vi "readFromXML.vi"(8 "error in (no error)":errorcluster, 10 "XML in":string, 11 "Ephemeris in":refnum<class "Ephemeris.lvclass">) -> (0 "error out":errorcluster, 3 "Ephemeris out":refnum<class "Ephemeris.lvclass">)   [LabVIEW 2022 SP3, in "TCSDataDefinitions.lvlib" / "TCSCommand.lvlib" / "TargetConfiguration.lvlib" / "Target.lvlib" / "Ephemeris.lvclass"]
uses:
  Ephemeris.lvclass
  Ephemeris.lvclass/Ephemeris.ctl
  Target/Target.lvclass
  <userlib>/Common/XML/XMLParser/XMLParser.lvclass
panel:
  out "file":string
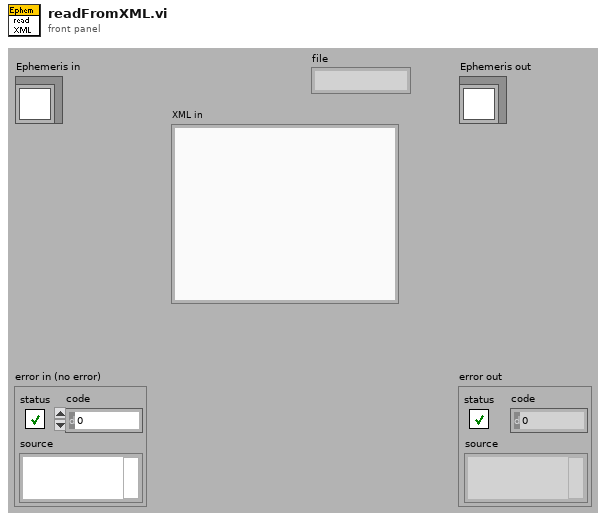
[diagram p1: front panel]
types:
  T1 = typedef "TCSDataDefinitions.lvlib/TCSCommand.lvlib/TargetConfiguration.lvlib/Target.lvlib/FixedTarget.lvlib/FrameValues.ctl" = enum16{"FK4", "FK5", "APPT", "GAPPT", "AZEL"}
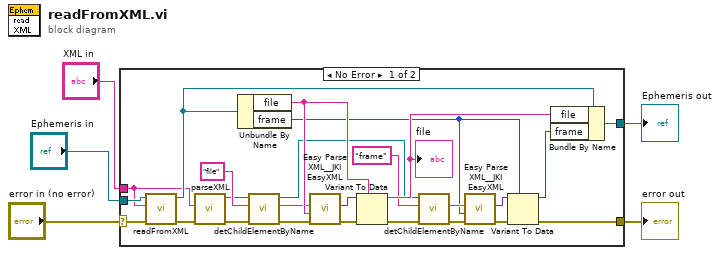
[diagram p0: block diagram]
diagram:
  n1 = case shown="No Error" "error in (no error)" {
    selector: "error in (no error)" -> [w23 w32]
    tunnel: [w6 w32] -> w4
    tunnel: [w26 w31] -> w2
    tunnel: "Ephemeris in" -> [w25 w31]
    tunnel: "XML in" -> [w21 _]
    frame No Error {
      n2 = call-parent "readFromXML.vi"("error in (no error)"=w23, "XML in"=w21, "Target in"=w25) -> ("error out"=w17:errorcluster, "Target out"=w24:refnum<class "Ephemeris.lvclass">)  [unwired: 7 in]
      n3 = call <userlib>:"parseXML.vi"("error in (no error)"=w17, "XMLString in"=w21) -> ("error out"=w22:errorcluster, "Element out"=w16:refnum<class "XMLParser.lvclass">)  [unwired: 8 in]
      n4 = Unbundle By Name(w24) -> ("file"=w28:string, "frame"=w9:T1)
      n5 = call <userlib>:"detChildElementByName.vi"("error in (no error)"=w22, "childName"="file" ("ChildName"), "Element in"=w16) -> ("error out"=w18:errorcluster, "childXML"=w19:string, "Element out"=w14:refnum<class "XMLParser.lvclass">)  [unwired: 5 in, 1 out]
      n6 = call <vilib>:"Easy Parse XML__JKI EasyXML.vi"("error in (no error)"=w18, "LabVIEW Data (Type)"=w28, "XML String"=w19) -> ("error out"=w29:errorcluster, "LabVIEW Data"=w30:variant)  [unwired: 7 out]
      n7 = Variant To Data(error in=w29, type=w28, Variant=w30) -> (data=w27:string, error out=w7:errorcluster)
      "file" <- w27
      n8 = call <userlib>:"detChildElementByName.vi"("error in (no error)"=w7, "childName"="frame", "Element in"=w14) -> ("error out"=w15:errorcluster, "childXML"=w12:string)  [unwired: 5 in, 2 out]
      n9 = call <vilib>:"Easy Parse XML__JKI EasyXML.vi"("error in (no error)"=w15, "LabVIEW Data (Type)"=w9, "XML String"=w12) -> ("error out"=w11:errorcluster, "LabVIEW Data"=w10:variant)  [unwired: 7 out]
      n10 = Variant To Data(error in=w11, type=w9, Variant=w10) -> (data=w8:T1, error out=w6:errorcluster)
      n11 = Bundle By Name(cluster=w24, "file"=w27, "frame"=w8) -> (w26:refnum<class "Ephemeris.lvclass">)
    }
    frame Error {
    }
  }
  "error out" <- w4
  "Ephemeris out" <- w2
